vi "Get channel servo info.vi"(8 "error in":errorcluster) -> (0 "error out":errorcluster, 1 "Cancelled":bool, 3 "Sampling info":T1={"Channels"=[], "Sampling freq"=0.0, "Output freq"=0.0, "Update freq"=0.0, "Steps per rev"=0, "Counts per rev"=0, "Amplifier"="", "Motor driver"="", "Step bit"=0, "Max speed"=0.0, "Max accel"=0.0, "Pos gain"=0.0, "Vel gain"=0.0, "counter"="Dev1/ctr0"} {"Channels"."Hi cutoff" items=["500"=500.0, "1k"=1000.0, "5k"=5000.0, "10k"=10000.0, "20k"=20000.0]; "Channels"."Lo cutoff" items=["0.1"=0.1, "1"=1.0, "10"=10.0, "100"=100.0, "300"=300.0]; "Channels"."Gain" items=["x100"=100, "x1000"=1000, "x10000"=10000]})   [LabVIEW 2013]
uses:
  Channel.ctl
  Sampling info.ctl
panel:
  in  "counter":tag="Dev1/ctr0" caption="Counter"
  in  "Pos gain in":dbl=1.0 caption="Position gain"
  in  "Max accel in":dbl[unit]=17453.292519943294 caption="Maximum acceleration"
  in  "Max speed in":dbl[unit]=87.26646259971648 caption="Maximum speed"
  in  "Output frequency in":dbl[unit]=50.0 caption="Output frequency"
  in  "Cancel":bool
  in  "OK":bool
  in  "Amplifier in":string(combo)="A-M Systems 1700" caption="Amplifier"
  in  "Update frequency in":dbl[unit]=20.0 caption="Update frequency"
  in  "Sampling frequency in":dbl[unit]=5000.0 caption="Sampling frequency"
  in  "Channels in":T2[](array[typedef]) caption="Channels" {"Hi cutoff" items=["500"=500.0, "1k"=1000.0, "5k"=5000.0, "10k"=10000.0, "20k"=20000.0]; "Lo cutoff" items=["0.1"=0.1, "1"=1.0, "10"=10.0, "100"=100.0, "300"=300.0]; "Gain" items=["x100"=100, "x1,000"=1000, "x10,000"=10000, "x100,000"=100000, "x1,000,000"=1000000]}
  # "Recording"
  # "Motor"
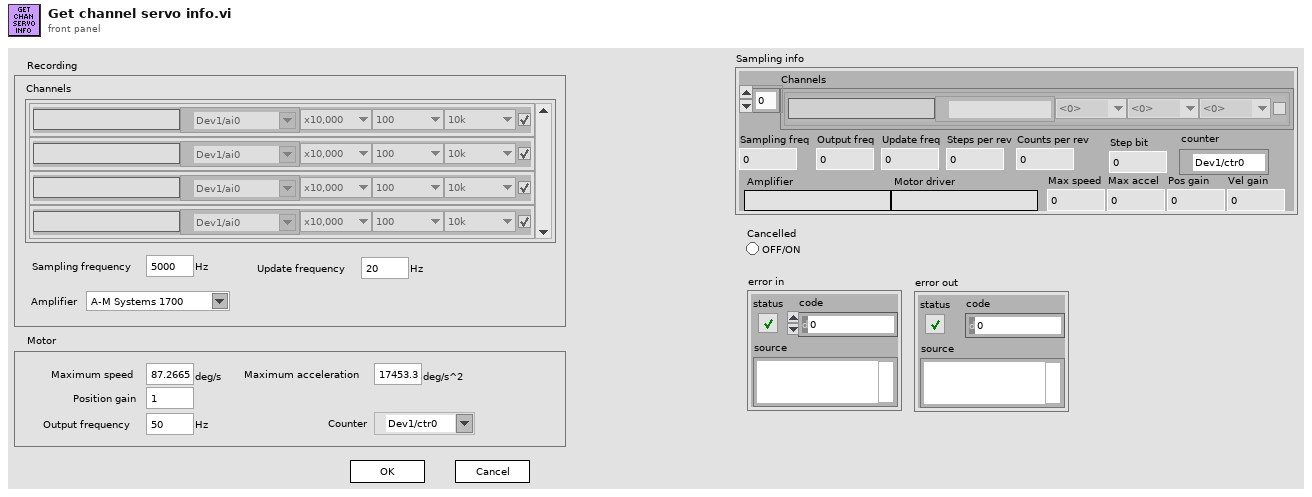
[diagram p1: front panel]
types:
  T1 = typedef "Sampling info.ctl" = cluster{"Channels":T2[], "Sampling freq":dbl, "Output freq":dbl, "Update freq":dbl, "Steps per rev":i32, "Counts per rev":i32, "Amplifier":string, "Motor driver":string, "Step bit":u8, "Max speed":dbl, "Max accel":dbl, "Pos gain":dbl, "Vel gain":dbl, "counter":tag}
  T2 = typedef "Channel.ctl" = cluster{"Name":string, "Chan":tag, "Gain":u32, "Lo cutoff":dbl, "Hi cutoff":dbl, "Notch":bool}
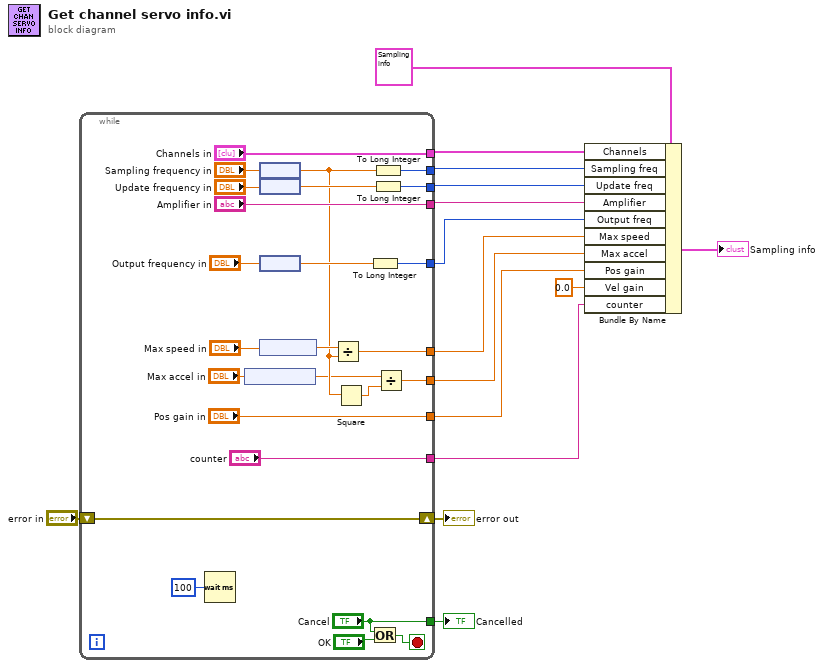
[diagram p0: block diagram]
diagram:
  n1 = while {
    tunnel: ["Cancel"] -> w8
    tunnel: ["Channels in"] -> w13
    tunnel: [w33] -> w14
    tunnel: [w32] -> w12
    tunnel: ["Amplifier in"] -> w11
    tunnel: [w27] -> w10
    shift-right: [w26] -> w6
    shift-left: "error in" -> [w26]
    tunnel: [w19] -> w5
    tunnel: [w18] -> w4
    tunnel: ["Pos gain in"] -> w3
    tunnel: ["counter"] -> w1
    stop <- w40 stop-if-true
    n2 = Wait (ms)(milliseconds to wait=u32 100) -> ()  [unwired: 1 out]
    n3 = node("Max accel in") -> (w20:dbl)
    n4 = node("Sampling frequency in") -> (w21:dbl)
    n5 = node("Update frequency in") -> (w30:dbl)
    n6 = node("Output frequency in") -> (w28:dbl)
    n7 = node("Max speed in") -> (w25:dbl)
    n8 = Divide(x=w25, y=w21) -> (x/y=w19:dbl)
    n9 = Square(x=w21) -> (x^2=w22:dbl)
    n10 = To Long Integer(number=w28) -> (32bit integer=w27:i32)
    n11 = Or(x="Cancel", y="OK") -> (x .or. y?=w40:bool)
    n12 = To Long Integer(number=w21) -> (32bit integer=w33:i32)
    n13 = To Long Integer(number=w30) -> (32bit integer=w32:i32)
    n14 = Divide(x=w20, y=w22) -> (x/y=w18:dbl)
  }
  "Cancelled" <- w8
  "error out" <- w6
  n15 = Bundle By Name(cluster=T1 {"Channels"=[], "Sampling freq"=0.0, "Output freq"=0.0, "Update freq"=0.0, "Steps per rev"=0, "Counts per rev"=0, "Amplifier"="", "Motor driver"="", "Step bit"=0, "Max speed"=0.0, "Max accel"=0.0, "Pos gain"=0.0, "Vel gain"=0.0, "counter"=""} ("Sampling data"), "Channels"=w13, "Sampling freq"=w14, "Update freq"=w12, "Amplifier"=w11, "Output freq"=w10, "Max speed"=w5, "Max accel"=w4, "Pos gain"=w3, "Vel gain"=0.0, "counter"=w1) -> (→"Sampling info":T1)
